vi "RemoveCrates.vi"(9 "From":i32, 10 "Qty":i32, 11 "StacksIn":string[][](array[string])) -> (2 "CratesRemoved":string[](array[string]), 3 "StacksOut":string[][](array[string]))   [LabVIEW 2020, in "2022_5.lvclass"]
uses:
  2022_5.lvclass
  1b76c4ed-dce1-40ab-9fd1-e0719c8f9599.vi
  1b76c4ed-dce1-40ab-9fd1-e0719c8f9599.vi/be6f088c-3e4b-4523-ad48-2cdc85bad38a.vi
  1b76c4ed-dce1-40ab-9fd1-e0719c8f9599.vi/f202eadf-433e-4cdb-b986-b2351ce8d73c.vi
  1b76c4ed-dce1-40ab-9fd1-e0719c8f9599.vi/094751bc-bcf2-4346-afae-53942128b536.vi
  2022_5.lvclass/2022_5.ctl
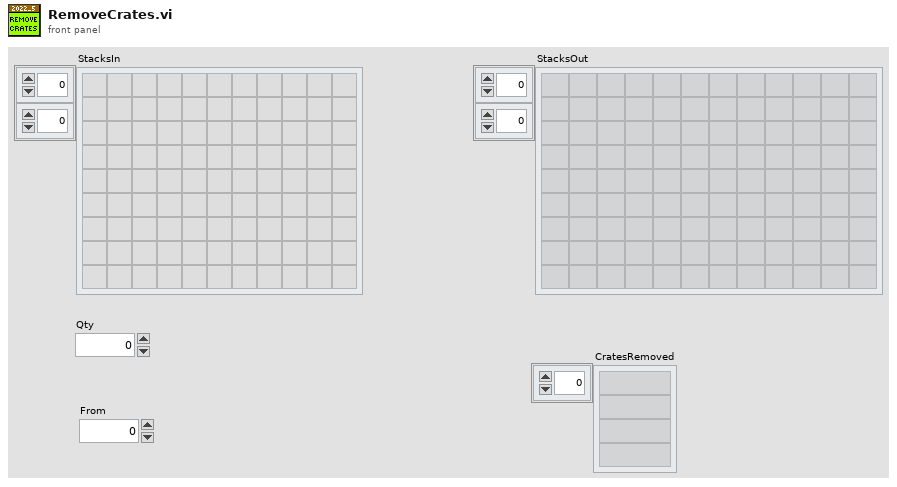
[diagram p1: front panel]
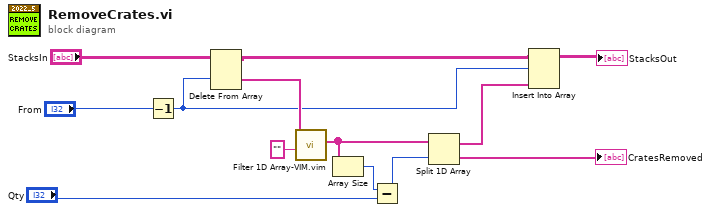
[diagram p0: block diagram]
diagram:
  n1 = Decrement(x="From") -> (x-1=w4:i32)
  n2 = Delete From Array(array="StacksIn", index (row)=w4) -> (deleted portion=w5:string[], array with subset deleted=w7:string[][])  [unwired: 2 in]
  n3 = call "Filter 1D Array-VIM.vim"("Item(s) to Filter"="", "Array"=w5) -> ("Filtered Array"=w11:string[])  [unwired: 5 in, 1 out]
  n4 = Array Size(array=w11) -> (size(s)=w2:i32)
  n5 = Subtract(x=w2, y="Qty") -> (x-y=w9:i32)
  n6 = Split 1D Array(array=w11, index=w9) -> (first subarray=w1:string[], second subarray=→"CratesRemoved":string[])
  n7 = Insert Into Array(array=w7, index (row)=w4, new element=w1) -> (→"StacksOut":string[][])  [unwired: 1 in]
